vi "test_CCDGetChipTemperature.vi"(7 "Test should pass":bool=TRUE, 8 "error in":errorcluster, 9 "tear down connection":bool=TRUE, 10 "set-up a connection":bool=TRUE, 11 "device selection":enum16{"monochromator", "CCD", "SCD"}(ring)=enum."CCD") -> (0 "error out":errorcluster)   [LabVIEW 2023]
uses:
  Source/Classes/Mono/Monochromator.lvclass
  Source/Classes/CCD/CCD.lvclass
  Source/Classes/SCD/SCD.lvclass
  <vilib>/addons/_JKI Toolkits/Caraya/classes/Assert/Assert Less_Variant.vi
  <vilib>/addons/_JKI Toolkits/Caraya/classes/Assert/Assert Greater_Variant.vi
  <vilib>/addons/_JKI Toolkits/Caraya/classes/Assert/Assert Not Error.vi
  <vilib>/addons/_JKI Toolkits/Caraya/classes/Assert/Assert Equal Type_Variant.vi
  Source/Classes/GenericDevice/GenericDevice.lvclass
  <vilib>/addons/_JKI Toolkits/Caraya/classes/Test/Test.lvclass
  <vilib>/addons/_JKI Toolkits/Caraya/classes/Assert/Assert.lvclass
panel:
  # "Connector Pane"
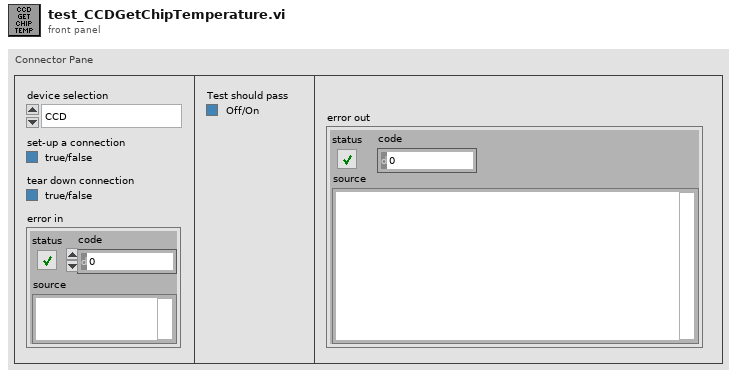
[diagram p1: front panel]
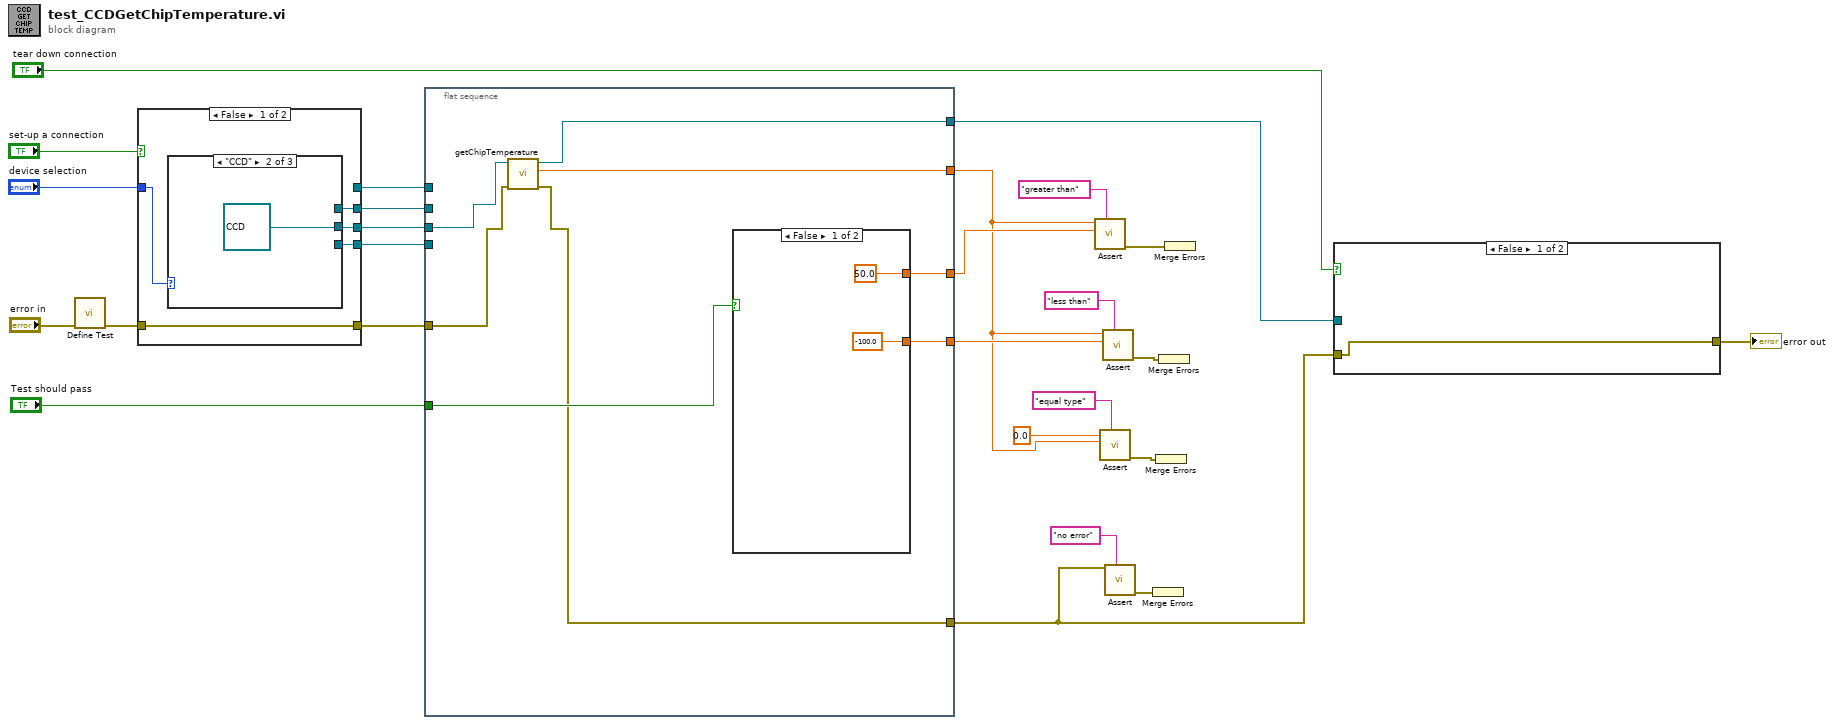
[diagram p0: block diagram]
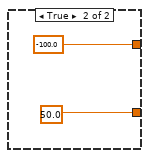
[diagram p2: hidden frame]
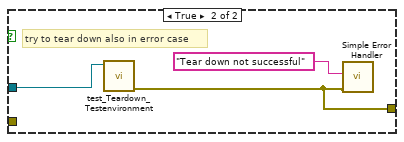
[diagram p3: hidden frame]
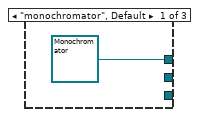
[diagram p4: hidden frame]
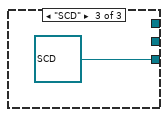
[diagram p5: hidden frame]
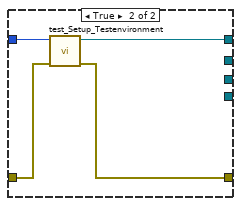
[diagram p6: hidden frame]
diagram:
  n1 = call <vilib>:"Define Test.vi"("error in (no error)"="error in") -> ("error out"=w18:errorcluster)  [unwired: 9 in, 1 out]
  n2 = case shown="False" "set-up a connection" {
    tunnel: w18 -> [w31 w38]
    tunnel: [w31 w37] -> w20
    tunnel: "device selection" -> [w30 w36]
    tunnel: [_ w35] -> w17
    tunnel: [w29 _] -> w16
    tunnel: [w28 _] -> w15
    tunnel: [w27 _] -> w14
    frame False {
      n3 = case shown="\"CCD\"" w30 {
        tunnel: [refnum<class "Monochromator.lvclass"> refnum ("Monochromator.lvclass") _ _] -> w29
        tunnel: [_ refnum<class "CCD.lvclass"> refnum ("CCD in") _] -> w28
        tunnel: [_ _ refnum<class "SCD.lvclass"> refnum ("SCD.lvclass")] -> w27
        frame "monochromator", Default {
        }
        frame "CCD" {
        }
        frame "SCD" {
        }
      }
    }
    frame True {
      n4 = call "test_Setup_Testenvironment.vi"("error in"=w38, "device selection"=w36) -> ("error out"=w37:errorcluster, "GenericDevice.lvclass"=w35:refnum<class "GenericDevice.lvclass">)  [unwired: 7 in, 1 out]
    }
  }
  n5 = flat-sequence {
    tunnel: w20 -> [w44]
    tunnel: w17 -> [_]
    tunnel: w16 -> [_]
    tunnel: w15 -> [w45]
    tunnel: w14 -> [_]
    tunnel: [w43] -> w9
    tunnel: "Test should pass" -> [w46]
    tunnel: [w42] -> w8
    tunnel: [w41] -> w2
    tunnel: [w40] -> w7
    tunnel: [w39] -> w6
    frame #0 {
      n6 = call "getChipTemperature.vi"("error in (no error)"=w44, "CCD in"=w45) -> ("error out"=w43:errorcluster, "temperature °C"=w41:dbl, "CCD out"=w42:refnum<class "CCD.lvclass">)  [unwired: 7 in]
      n7 = case shown="False" w46 {
        tunnel: [50.0 ("temperature °C") -100.0 ("temperature °C")] -> w40
        tunnel: [-100.0 ("temperature °C") 50.0 ("temperature °C")] -> w39
        frame False {
          (unwired) 255
          (unwired) 1023
        }
        frame True {
        }
      }
    }
  }
  n8 = call-poly <vilib>:"Assert.vi"("Label"="greater than" ("Label (VI Title)"), "Y"=w7, "X"=w2) -> ("error out"=w24:errorcluster)  [unwired: 7 in, 1 out]
  n9 = call-poly <vilib>:"Assert.vi"("Label"="equal type" ("Label (VI Title)"), "Y"=w2, "X"=0.0 ("temperature °C")) -> ("error out"=w4:errorcluster)  [unwired: 7 in, 1 out]
  n10 = call-poly <vilib>:"Assert.vi"("Label"="less than" ("Label (VI Title)"), "Y"=w6, "X"=w2) -> ("error out"=w22:errorcluster)  [unwired: 7 in, 1 out]
  n11 = call-poly <vilib>:"Assert.vi"("Label"="no error" ("Label (VI Title)"), "Not Error?"=w9) -> ("error out"=w11:errorcluster)  [unwired: 8 in, 1 out]
  n12 = Merge Errors(w11) -> ()  [unwired: 1 out]
  n13 = Merge Errors(w4) -> ()  [unwired: 1 out]
  n14 = Merge Errors(w22) -> ()  [unwired: 1 out]
  n15 = Merge Errors(w24) -> ()  [unwired: 1 out]
  n16 = case shown="False" "tear down connection" {
    tunnel: w8 -> [_ w53]
    tunnel: [w51 w52] -> w1
    tunnel: w9 -> [w51 _]
    frame False {
    }
    frame True {
      # "try to tear down also in error case"
      n17 = call "test_Teardown_Testenvironment.vi"("GenericDevice.lvclass"=w53) -> ("error out"=w52:errorcluster)  [unwired: 9 in, 1 out]
      n18 = call <vilib>:"Simple Error Handler.vi"("error source (\" \")"="Tear down not successful" ("error source (\" \")"), "error in (no error)"=w52) -> ()  [unwired: 3 in, 5 out]
    }
  }
  "error out" <- w1
